vi "Create.vi"(3 "Parent Name":string) -> (1 "Logger Identity out":refnum<class "Logger Identity.lvclass">)   [LabVIEW 2020, in "VolatusData.lvlib" / "Logger Identity.lvclass"]
uses:
  Logger Identity.lvclass
  Logger Identity.lvclass/Logger Identity.ctl
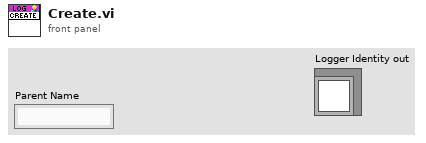
[diagram p1: front panel]
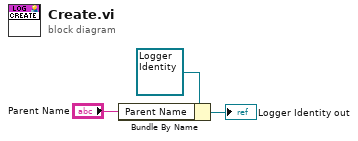
[diagram p0: block diagram]
diagram:
  n1 = Bundle By Name(cluster=refnum<class "Logger Identity.lvclass"> refnum ("DataProc Identity in"), "Parent Name"="Parent Name") -> (→"Logger Identity out":refnum<class "Logger Identity.lvclass">)
